vi "Main.vi"   [LabVIEW 2020]
uses:
  Actor/Nested/Nested.lvclass
  C:/Program Files/National Instruments/LabVIEW 2020/vi.lib/ActorFramework/Actor/Actor.lvclass
  <vilib>/ActorFramework/Actor/Actor.lvclass
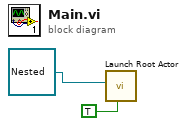
[diagram p0: block diagram]
diagram:
  n1 = call <vilib>:"Launch Root Actor.vi"("Open Actor Core front panel? (F)"=TRUE, "Actor"=refnum<class "Nested.lvclass"> refnum ("Nested.lvlib:Nested.lvclass")) -> ()  [unwired: 8 in, 2 out]
